vi "Set Encoder Position [LCP].vi"(7 "Micropulse # In":i32, 8 "error in (no error)":errorcluster, 10 "Position (mm)":dbl=1.0 max=255.0, 11 "Axis No.":u8=1 min=1 max=4) -> (0 "error out":errorcluster, 5 "Micropulse # Out":i32)   [LabVIEW 2026, in "MicroPulse_Driver.lvlib"]
doc: "This command allows the global setting of encoder parameters. Mode 0 is the default mode of 24-bit encoders with the standard output message format. Mode 1 is the full 32-bit output mode. In mode 2 the output mode is full 32 bit but also the output message of inspection modes FLR and FLX/FLZ are now a 32-bit LLC message giving all axis positions instead of the normal LCI message that only gave information about a single axis. Further modes are available 3, 4, and 5 that give the same as modes 0, 1 and 2 but also include with the axis data a message that gives the status of the input/output lines. This message is the same as the reply to an STS 6 command.\n\nThe input mode and filter count are optional parameters. The input mode sets all axis as either full Quadrature or Step/Direction. In Step/Direction the ‘A+’ input is the Step whilst the ‘B+’ is the Direction. Each complete Step pulse is two encoder counts. The filter count is a parameter that can used to clean up the edges of noisy encoders by time hysteresis. This defines the length of time before a decision is made on any input transitions and can filter out noise spikes and noisy level transitions.\nFor individual setting of the Input Mode and Filter Count see the ENCT and ENCF command respectively. It is recommended that these are used.\n\nThe optional fourth parameter (LLC Freq) allows the setting of an increased number of LLC messages (as defined by the Mode parameter above). Normally only one LLC is sent at the start of a data set. If this parameter is used then an LLC will be still sent at the start of a data set, but then further LLC messages will be sent during the data set on before every nth test.\n\nParameters:\n<Mode> : Integer value from 0 to 5:\n0 = 24 Bit output (Default)\n1 = 32 Bit output\n2 = 32 Bit output with LLC message for moving inspection modes\n3 = 24 Bit output with STS 6 message\n4 = 32 Bit output with STS 6 message\n5 = 32 Bit output with LLC message for moving inspection modes with STS 6 message\n\n[Input Mode] : Integer 0 or 1:\n0 = Quadrature (Default)\n1 = Step/Direction\n\n[Filter Count] : Integer value from 0 to 255:\n0 = OFF (Default 0)\n1 to 255 = approximately 100nSec to 20uSec\n\n[LLC Freq] : Integer value \"n\" from 0 to 100 (default 0).\n\nNote:\nThe 32-bit encoders require longer messages for LLC, LCI and LCA. The format is shown in the MicroPulse Output Messages Section.\n\nSystem Compatibility:\nLT1 supports only mode 0 – 2"
uses:
  MicroPulse_Driver.lvlib
  Private/MP-Registry Action-Enum.ctl
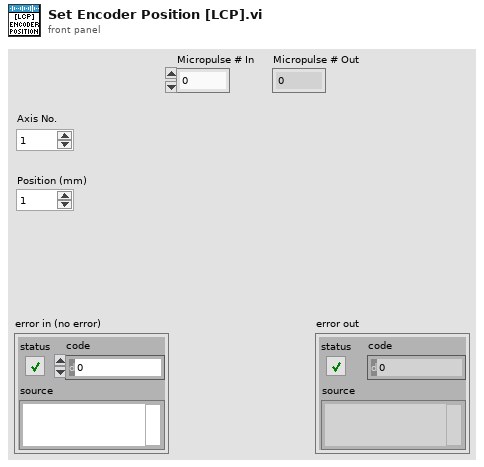
[diagram p1: front panel]
types:
  T1 = typedef "MicroPulse_Driver.lvlib/MP-Registry Action-Enum.ctl" = enum16{"Read", "Add Test", "Add Command", "Add Gate Command", "Add Encoder Command", "Clear Command  List", "Set Registry", "Set System Details", "Set DOF", "Set Velocity", "Disable Asynch Reads", "Enable Asynch Reads", "Add Connection", "Disconnect", "Shutdown"}
  T2 = typedef "MicroPulse_Driver.lvlib/MP-Registry Data-Cluster.ctl" = cluster{"Instrument Type":T3, "Serial #":u64, "Sample Frequency":T4, "dt (us)":dbl, "DOF":T5, "Material Velocity":dbl, "Asynch Reads":T6, "NUM of Tests":u32, "System Details":T7, "Gates":T9[], "Encoders":T16[], "CMD LUT":variant, "Command List":string}
  T3 = typedef "MicroPulse_Driver.lvlib/MP - instrument type.ctl" = enum16{"MicroPulse 5", "LT1", "LT2", "LTPA", "MPLT", "MicroPulse 6", "PipeScanner", "<MicroPulse>", "Micropulse 4", "Simulated Data"}
  T4 = typedef "MicroPulse_Driver.lvlib/MP - sample frequency.ctl" = enum16{"Use Default", "200MHz (LT2 only)", "100MHz", "50MHz", "25MHz", "10MHz"}
  T5 = typedef "MicroPulse_Driver.lvlib/MP - data output format.ctl" = enum16{"", "8-bit Mode", "10-bit Mode", "12-bit Mode", "16-bit Mode", "8-bit Log Mode", "12-bit Packed Mode"}
  T6 = typedef "MicroPulse_Driver.lvlib/MP - asynch read mode.ctl" = enum16{"Disabled", "Enabled"}
  T7 = typedef "MicroPulse_Driver.lvlib/MP - general system status.ctl" = cluster{"System Type":T3, "Serial No.":u64, "Channels":cluster{"Conv":u8, "PA":u16, "Extra":u32}, "Sample Frequency":cluster{"Default":u8, "Actual":u8}, "Software Versions":string, "Data Output Format":cluster{"Default":T5, "Actual":T5}, "Temperatures":cluster{"System":u8, "Processor":u8, "Slave Sys":u8, "Slave Proc":u8}, "Tx Buffer Size":u32, "System Error":string, "No. of Cards":u8, "DAC Gain":i16, "Uptimes":cluster{"since Power":u32, "since RSTS":u32, "since SRST":u32}, "Voltages":cluster{"Nominal":dbl, "Measured":dbl, "Difference":dbl}[], "Interface Cards":T8[]}
  T8 = typedef "MicroPulse_Driver.lvlib/MP - interface card status.ctl" = cluster{"Status":u8, "Map":u8, "Board - T":u8, "FPGA - T":u8, "PAIF Status":string, "Version":string}
  T9 = typedef "MicroPulse_Driver.lvlib/MP - Registry Gates.ctl" = cluster{"Display Gate":T10, "ETM Mode":T11, "Echo Gate":T12, "Insp Gates":T13[]}
  T10 = typedef "MicroPulse_Driver.lvlib/MP - display gate.ctl" = cluster{"Start":dbl, "Length":dbl}
  T11 = typedef "MicroPulse_Driver.lvlib/MP - echo gate mode.ctl" = enum16{"Echo Trigger OFF", "Echo Gate Display Mode", "Echo Trigger ON", "Multi Gate or FMC Mode", "Reserved", "PA - Echo Trigger ON"}
  T12 = typedef "MicroPulse_Driver.lvlib/MP - echo gate parameters.ctl" = cluster{"Start (us)":dbl, "Length (us)":dbl, "Threshold":u16, "Colour":u32}
  T13 = typedef "MicroPulse_Driver.lvlib/MP - multigate inspection gate parameters.ctl" = cluster{"Start (us)":dbl, "Length (us)":dbl, "Threshold":u16, "Enabled?":bool, "Max # Peaks":u16, "Hysteresis":T14, "Mode":T15, "Inverted?":bool, "Colour ":u32}
  T14 = typedef "MicroPulse_Driver.lvlib/MP - hysteresis level.ctl" = enum16{"None", "3dB", "6dB", "9dB", "12dB"}
  T15 = typedef "MicroPulse_Driver.lvlib/MP - multigate mode.ctl" = enum16{"1st Peak in Gate", "Largest Peak In Gate", "All Peaks In Gate", "1st Threshold Crossing"}
  T16 = typedef "MicroPulse_Driver.lvlib/MP - encoder settings.ctl" = cluster{"Encoder Type":T17, "Counts/mm":u32, "Enable Termination?":bool, "Multiplier":u32, "Backlash Period (s)":dbl, "Encoder Filter":u32}
  T17 = typedef "MicroPulse_Driver.lvlib/MP - encoder type.ctl" = enum16{"Quadrature", "Step/Direction"}
  T18 = typedef "MicroPulse_Driver.lvlib/TCP config.ctl" = cluster{"Connection ID":refnum<k5>, "IP address":string, "host port":u16, "OC timeout":i32, "Read timeout":i32, "Write timeout":i32}
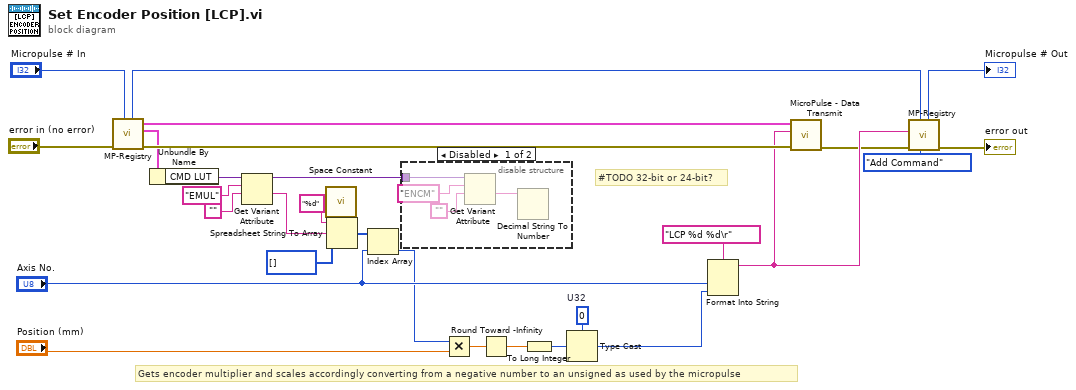
[diagram p0: block diagram]
diagram:
  w2 = u32 0  # U32
  # "#TODO 32-bit or 24-bit?"
  # "Gets encoder multiplier and scales accordingly converting from a negative number to an unsigned as used by the micropulse"
  n1 = call "MP-Registry.vi"("Micropulse # In"="Micropulse # In", "error in (no error)"="error in (no error)") -> ("error out"=w27:errorcluster, "Micropulse Data"=w18:T2, "TCP config"=w26:T18, "Micropulse # Out"=w22:i32)  [unwired: 6 in]
  n2 = Unbundle By Name(w18) -> ("CMD LUT"=w17:variant)
  n3 = Get Variant Attribute(Variant=w17, name="EMUL", default value (empty Variant)="") -> (duplicate Variant=w1:variant, value=w14:string)  [unwired: 1 in, 2 out]
  n4 = call <vilib>:"Space Constant.vi"() -> ("String"=w10:string)
  n5 = Spreadsheet String To Array(delimiter (Tab)=w10, format string="%d", spreadsheet string=w14, array type (2D Dbl)=i32[] []) -> (array=w12:i32[])
  n6 = Index Array(array=w12, index="Axis No.") -> (element=w8:i32)
  n7 = disable-structure shown="Disabled" {
    disable-tunnel: w1 -> [w33 _]
    frame Disabled {
      n8 = Get Variant Attribute(Variant=w33, name="ENCM", default value (empty Variant)="") -> (value=w30:string)  [unwired: 1 in, 3 out]
      n9 = Decimal String To Number(string=w30) -> ()  [unwired: 2 in, 2 out]
    }
    frame Enabled {
    }
  }
  n10 = Multiply(x=w8, y="Position (mm)") -> (x*y=w6:dbl)
  n11 = Round Toward -Infinity(1:w6) -> (0:w5:dbl)
  n12 = To Long Integer(number=w5) -> (32bit integer=w4:i32)
  n13 = Type Cast(type=w2, x=w4) -> (*(type *) &x=w3:u32)
  n14 = Format Into String(format string="LCP %d %d\r", "Axis No.", w3) -> (resulting string=w25:string)  [unwired: 2 in, 1 out]
  n15 = call "MicroPulse - Data Transmit.vi"("error in (no error)"=w27, "data"=w25, "TCP config"=w26) -> ("error out"=w23:errorcluster)  [unwired: 6 in, 2 out]
  n16 = call "MP-Registry.vi"("Action"=MP-Registry_Action-Enum."Add Command", "Micropulse # In"=w22, "error in (no error)"=w23, "Data in"=w25) -> ("error out"=→"error out":errorcluster, "Micropulse # Out"=→"Micropulse # Out":i32)  [unwired: 4 in, 2 out]
